vi "递规测试.vi"(8 "数值":i32, 11 "数组":i32[](array[numeric])) -> (3 "数组 2":i32[](array[numeric]))   [LabVIEW 2018]
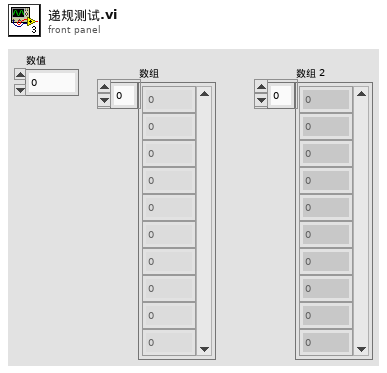
[diagram p1: front panel]
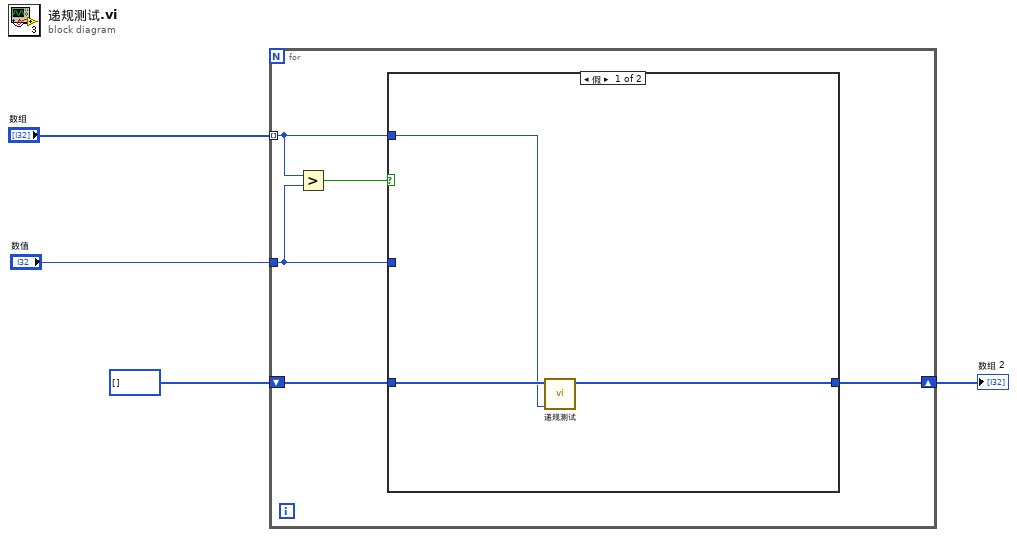
[diagram p0: block diagram]
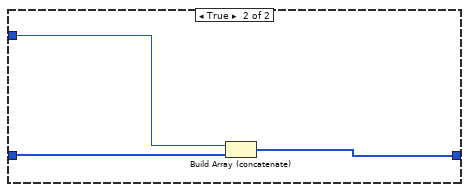
[diagram p2: hidden frame]
diagram:
  n1 = for {
    tunnel: "数组" -> [w5] mode=indexing
    tunnel: "数值" -> [w7]
    shift-right: [w6] -> w1
    shift-left: i32[] [] ("数组") -> [w8]
    n2 = Greater?(x=w5, y=w7) -> (0:w9:bool)
    n3 = case shown="假" w9 {
      tunnel: w8 -> [w12 w15]
      tunnel: w7 -> [_ w14]
      tunnel: [w11 w13] -> w6
      tunnel: w5 -> [w10 _]
      frame False {
        n4 = call "递规测试.vi"("数值"=w10, "数组"=w12) -> ("数组 2"=w11:i32[])  [unwired: 9 in]
      }
      frame True {
        n5 = Build Array (concatenate)(w14, w15) -> (w13:i32[])
      }
    }
  }
  "数组 2" <- w1
